vi "图片颜色识别.vi"() -> ()   [LabVIEW 2018]
uses:
  <vilib>/vision/NI_Vision_Development_Module.lvlib
panel:
  out "FoundYellow":bool
  out "FoundGreen":bool
  out "FoundRed":bool
  in  "error in (no error)":errorcluster
  out "error out":errorcluster
  in  "停止":bool
  out "Color Spectrum":dbl[](array[numeric]) format="%.2f"
  in  "Rectangle":T1 {"Rotation" min=-90.0 max=90.0 step=1.0 format="%.2f"; "Left" scale=0.0..1024.0; "Right" scale=0.0..1024.0}
  in  "File Path":path
  out "Image":T2(plugin-control)
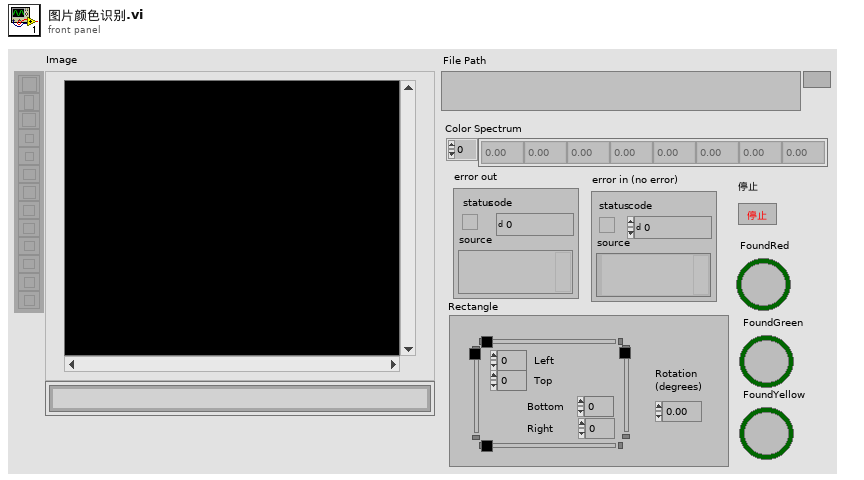
[diagram p1: front panel]
types:
  T1 = typedef "IMAQ Rectangle" = cluster{"Left":i32, "Top":i32, "Right":i32, "Bottom":i32, "Rotation":dbl}
  T2 = typedef "IMAQ Image.ctl" = refnum<image>
  T3 = typedef "ROI Descriptor" = cluster{"Global Rectangle":i32[], "Contours":cluster{"ID":enum32{"External", "Internal"}, "Type":u32, "Coordinates":i32[]}[]}
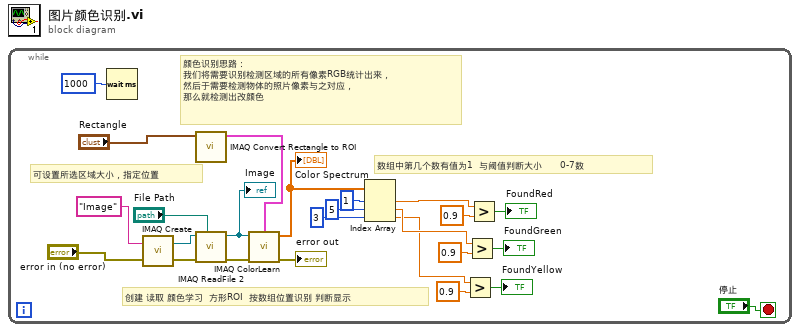
[diagram p0: block diagram]
diagram:
  n1 = while {
    stop <- "停止" stop-if-true
    # "创建 读取 颜色学习  方形ROI  按数组位置识别 判断显示"
    # "可设置所选区域大小，指定位置"
    # "数组中第几个数有值为1  与阈值判断大小      0-7数"
    # "颜色识别思路：\n我们将需要识别检测区域的所有像素RGB统计出来，\n然后于需要检测物体的照片像素与之对应，\n那么就检测出改颜色"
    n2 = Wait (ms)(milliseconds to wait=u32 1000 ("等待时间（毫秒）")) -> ()  [unwired: 1 out]
    n3 = call "IMAQ Create"("Image Name"="Image", "error in (no error)"="error in (no error)") -> ("New Image"=w25:T2, "error out"=w24:errorcluster)  [unwired: 3 in]
    n4 = call "IMAQ Convert Rectangle to ROI"("Rectangle"="Rectangle") -> ("ROI Descriptor"=w19:T3)  [unwired: 8 in, 1 out]
    n5 = call "IMAQ ReadFile 2"("File Path"="File Path", "error in (no error)"=w24, "Image"=w25) -> ("error out"=w20:errorcluster, "Image Out"=w21:T2)  [unwired: 4 in, 3 out]
    "Image" <- w21
    n6 = call "IMAQ ColorLearn"("ROI Descriptor"=w19, "Image"=w21, "error in (no error)"=w20) -> ("Color Spectrum"=w13:dbl[], "error out"=→"error out":errorcluster)  [unwired: 5 in]
    "Color Spectrum" <- w13
    n7 = Index Array(array=w13, index #1=1 ("索引"), index #2=5 ("索引"), index #3=3 ("索引")) -> (element #1=w11:dbl, element #2=w5:dbl, element #3=w1:dbl)
    n8 = Greater?(x=w1, y=0.9) -> (0:→"FoundYellow":bool)
    n9 = Greater?(x=w5, y=0.9) -> (0:→"FoundGreen":bool)
    n10 = Greater?(x=w11, y=0.9) -> (0:→"FoundRed":bool)
  }
